vi "InsertSearch.vi"(10 "EventQueue":T2(array[cluster]), 11 "Event":T3) -> (3 "Index":i32)   [LabVIEW 2014]
uses:
  TypeDefs/Point2D.ctl
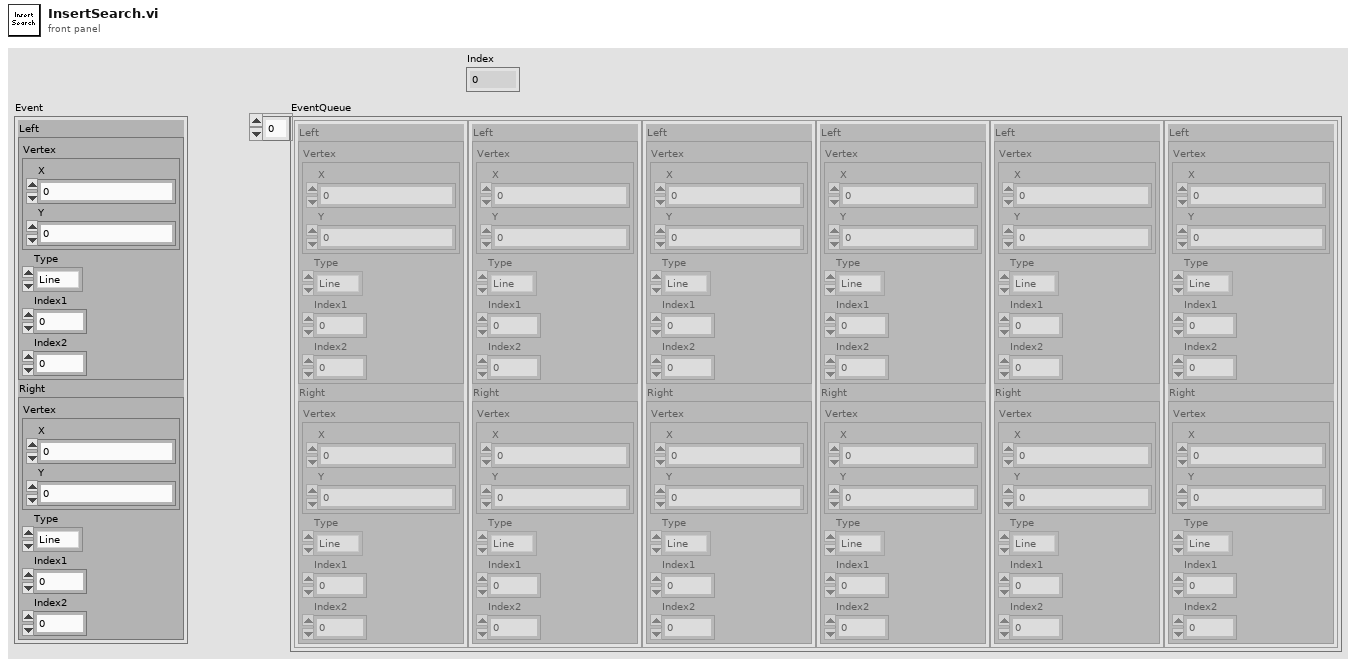
[diagram p1: front panel]
types:
  T1 = typedef "Point2D.ctl" = cluster{"X":sgl, "Y":sgl}
  T2 = cluster{"Left":cluster{"Vertex":T1, "Type":enum16{"Line", "Poly", "Cross"}, "Index1":i32, "Index2":i32}, "Right":cluster{"Vertex":T1, "Type":enum16{"Line", "Poly", "Cross"}, "Index1":i32, "Index2":i32}}[]
  T3 = cluster{"Left":cluster{"Vertex":T1, "Type":enum16{"Line", "Poly", "Cross"}, "Index1":i32, "Index2":i32}, "Right":cluster{"Vertex":T1, "Type":enum16{"Line", "Poly", "Cross"}, "Index1":i32, "Index2":i32}}
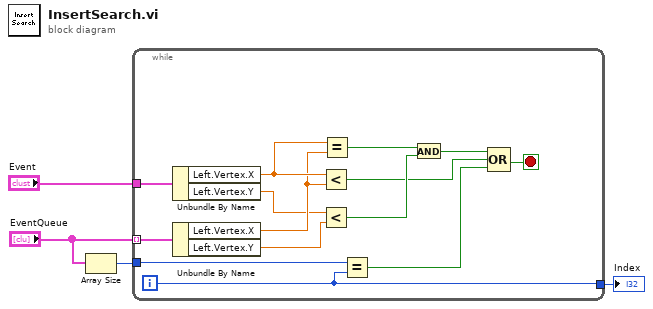
[diagram p0: block diagram]
diagram:
  n1 = Array Size(array="EventQueue") -> (size(s)=w1:i32)
  n2 = while {
    tunnel: "EventQueue" -> [w17] mode=indexing
    tunnel: "Event" -> [w18]
    tunnel: [w9] -> w3
    tunnel: w1 -> [w10]
    i -> [w9]
    stop <- w8 stop-if-true
    n3 = Unbundle By Name(w18) -> ("Left.Vertex.X"=w16:sgl, "Left.Vertex.Y"=w14:sgl)
    n4 = Unbundle By Name(w17) -> ("Left.Vertex.X"=w15:sgl, "Left.Vertex.Y"=w13:sgl)
    n5 = Less?(x=w16, y=w15) -> (x < y?=w6:bool)
    n6 = Less?(x=w14, y=w13) -> (x < y?=w11:bool)
    n7 = Equal?(x=w16, y=w15) -> (x = y?=w12:bool)
    n8 = Equal?(x=w10, y=w9) -> (x = y?=w5:bool)
    n9 = And(x=w12, y=w11) -> (x .and. y?=w7:bool)
    n10 = Compound Arithmetic op=OR(w7, w6, w5) -> (w8:bool)
  }
  "Index" <- w3
